vi "valve_shaking - Copy.vi"(0 "Z":T3={"Z_ASw"=1, "Z_HSetState"=enum."on", "Z_ASetState"=enum."on", "Z_DSetState"=enum."on"}, 5 "Y":T1={"Y_ASw"=1, "Y_HSetState"=enum."auto", "Y_ASetState"=enum."auto", "Y_DSetState"=enum."auto"}, 9 "ALR_DI":T2, 12 "Parameters table":u32[](array[numeric])=[0, 10000, 100, 5000, 100, 5000, 1000, 3000]) -> (4 "Z_out":T4, 6 "YB":bool[](array[boolean]), 10 "ALR_ON":bool[](array[boolean]))   [LabVIEW 2015]
uses:
  Userlib.lvlib
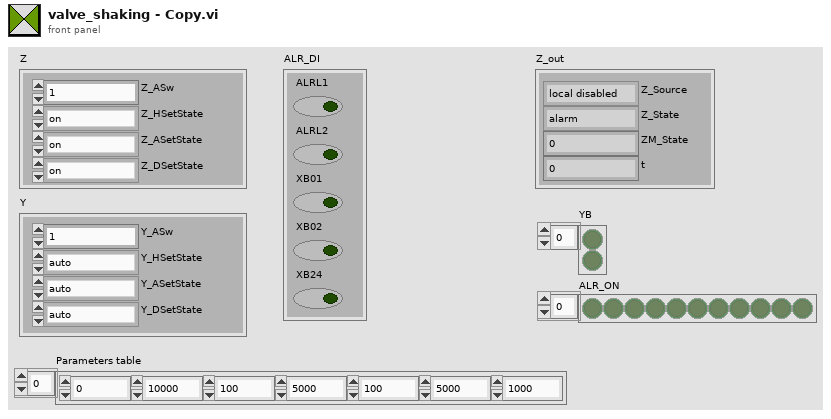
[diagram p1: front panel]
types:
  T1 = cluster{"Y_ASw":u32, "Y_HSetState":enum8{"alarm", "min", "stop", "hand", "auto", "max"}, "Y_ASetState":enum8{"alarm", "min", "stop", "hand", "auto", "max"}, "Y_DSetState":enum8{"alarm", "min", "stop", "hand", "auto", "max"}}
  T2 = cluster{"ALRL1":bool, "ALRL2":bool, "XB01":bool, "XB02":bool, "XB24":bool}
  T3 = cluster{"Z_ASw":u32, "Z_HSetState":enum8{"alarm", "disabled", "not ready", "stop ready", "reserv", "switched off", "switched on", "check", "on min", "decrease speed", "on", "increase speed", "on max"}, "Z_ASetState":enum8{"alarm", "disabled", "not ready", "stop ready", "reserv", "switched off", "switched on", "check", "on min", "decrease speed", "on", "increase speed", "on max"}, "Z_DSetState":enum8{"alarm", "disabled", "not ready", "stop ready", "reserv", "switched off", "switched on", "check", "on min", "decrease speed", "on", "increase speed", "on max"}}
  T4 = cluster{"Z_Source":enum8{"local disabled", "local hand", "hand", "auto", "dist"}, "Z_State":enum8{"alarm", "disabled", "not ready", "stop ready", "reserv", "switched off", "switched on", "check", "on min", "decrease speed", "on", "increase speed", "on max"}, "ZM_State":u8, "t":u32}
  T5 = enum8{"alarm", "disabled", "not ready", "stop ready", "reserv", "switched off", "switched on", "check", "on min", "decrease speed", "on", "increase speed", "on max"}
  T6 = enum8{"local disabled", "local hand", "hand", "auto", "dist"}
  T7 = cluster{"Z_Source_Out":enum8{"local disabled", "local hand", "hand", "auto", "dist"}, "Z_State":enum8{"alarm", "disabled", "not ready", "stop ready", "reserv", "switched off", "switched on", "check", "on min", "decrease speed", "on", "increase speed", "on max"}, "ZM_State":u32, "t":u32}
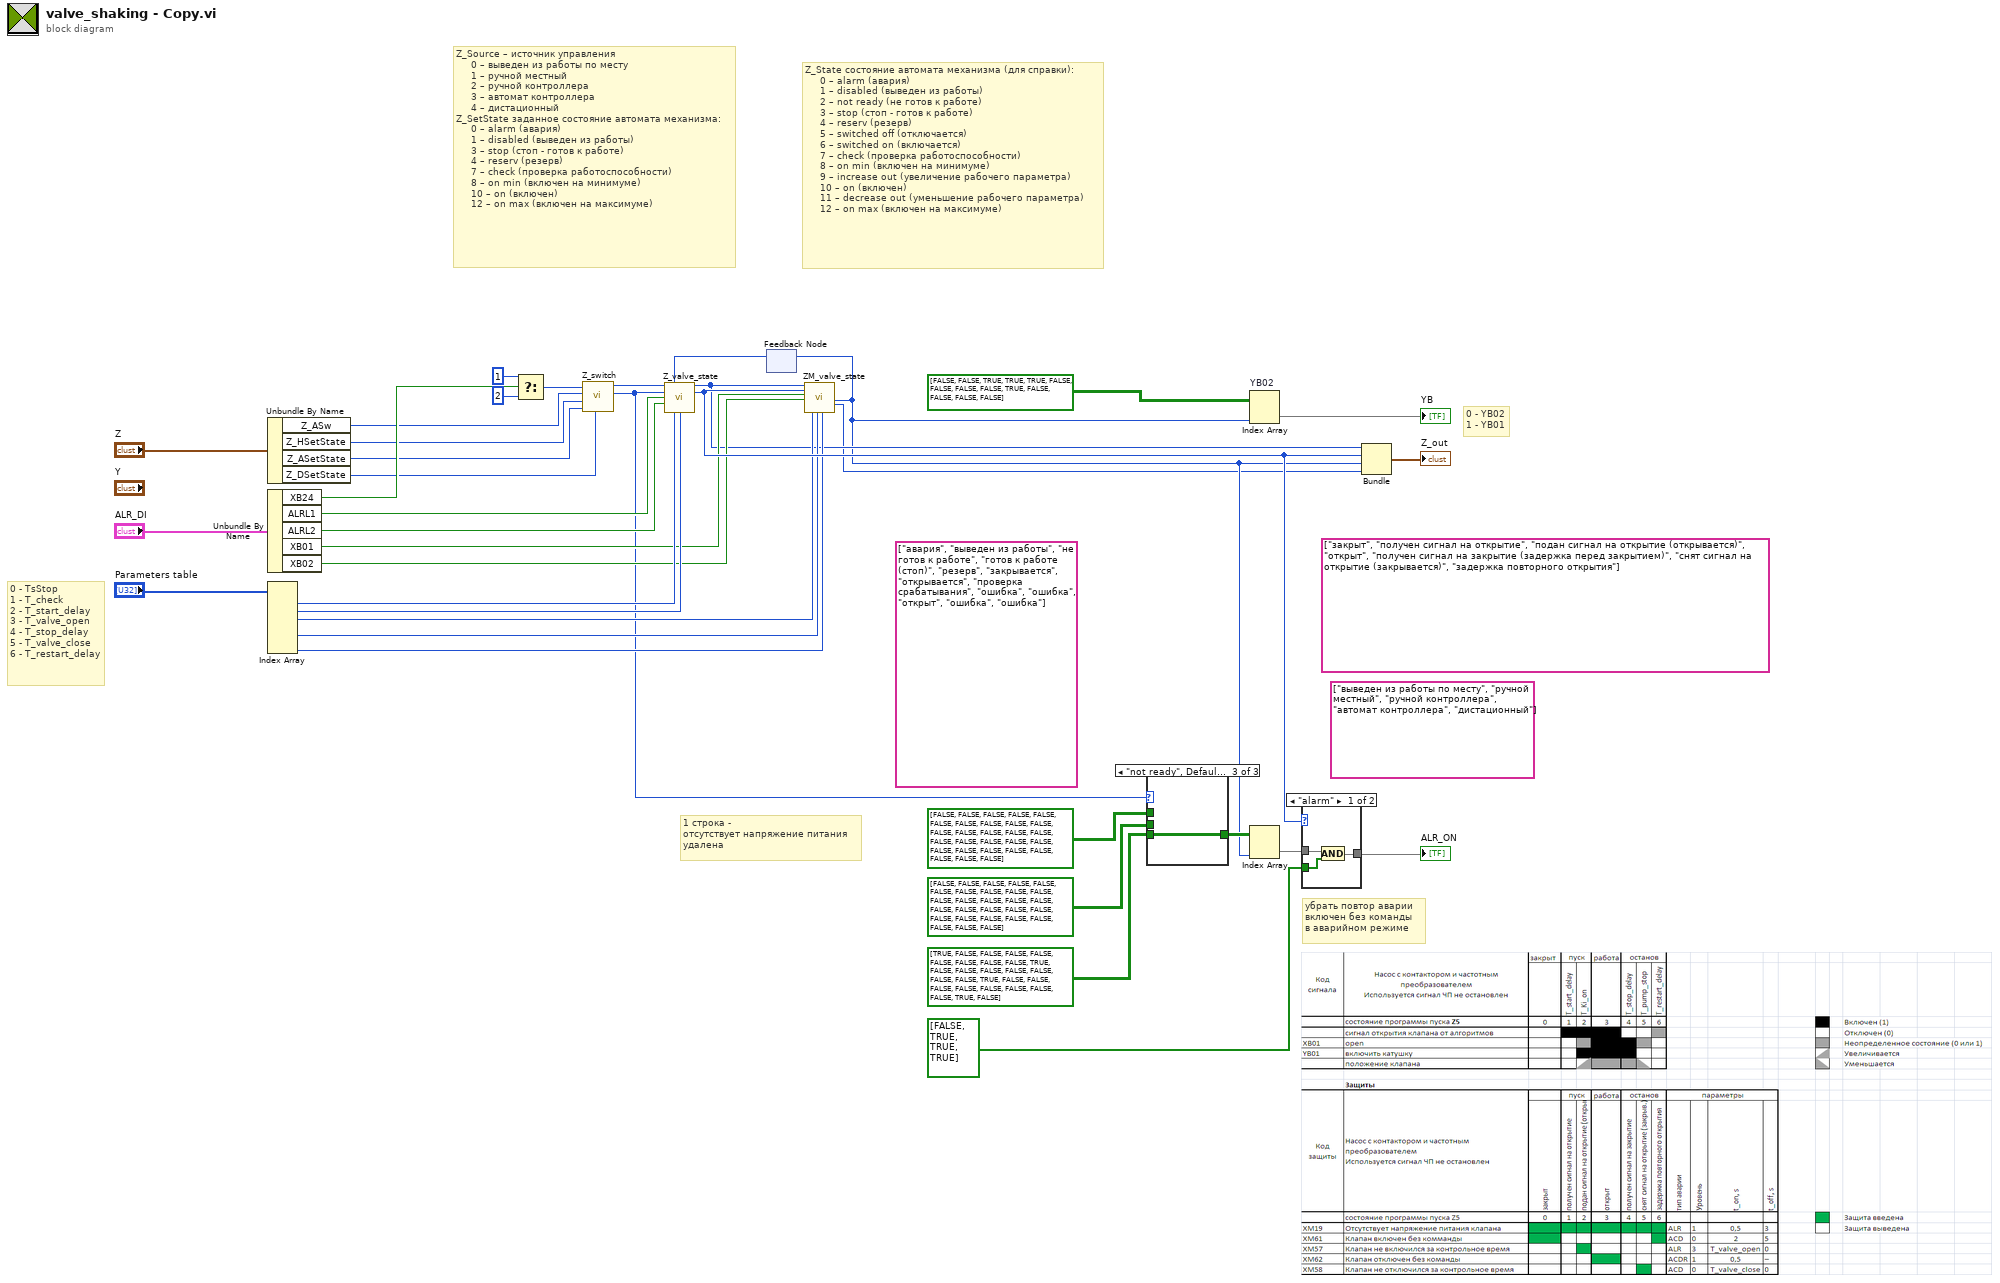
[diagram p0: block diagram]
diagram:
  (unwired) string[] ["закрыт", "получен сигнал на открытие", "подан сигнал на открытие (открывается)", "открыт", "получен сигнал на закрытие (задержка перед закрытием)", "снят сигнал на открытие (закрывается)", "задержка повторного открытия"]
  (unwired) string[] ["выведен из работы по месту", "ручной местный", "ручной контроллера", "автомат контроллера", "дистационный"]
  (unwired) string[] ["авария", "выведен из работы", "не готов к работе", "готов к работе (стоп)", "резерв", "закрывается", "открывается", "проверка срабатывания", "ошибка", "ошибка", "открыт", "ошибка", "ошибка"]
  # "0 - YB02\n1 - YB01"
  # "1 строка - \nотсутствует напряжение питания\nудалена"
  # "убрать повтор аварии\nвключен без команды\nв аварийном режиме"
  # "0 - TsStop\n1 - T_check\n2 - T_start_delay\n3 - T_valve_open\n4 - T_stop_delay\n5 - T_valve_close\n6 - T_restart_delay"
  # "Z_Source – источник управления\n     0 – выведен из работы по месту\n     1 – ручной местный\n     2 – ручной контроллера\n     3 – автомат контроллера\n     4 – дистационный\nZ_SetState заданное состояние автомата механизма:\n     0 – alarm (авария)\n     1 – disabled (выведен из работы)\n     3 – stop (стоп - готов к работе)\n     4 – reserv (резерв)\n     7 – check (проверка работоспособности)\n     8 – on min (включен на минимуме)\n     10 – on (включен)\n     12 – on max (включен на максимуме)"
  # "Z_State состояние автомата механизма (для справки):\n     0 – alarm (авария)\n     1 – disabled (выведен из работы)\n     2 – not ready (не готов к работе)\n     3 – stop (стоп - готов к работе)\n     4 – reserv (резерв)\n     5 – switched off (отключается)\n     6 – switched on (включается)\n     7 – check (проверка работоспособности)\n     8 – on min (включен на минимуме)\n     9 – increase out (увеличение рабочего параметра)\n     10 – on (включен)\n     11 – decrease out (уменьшение рабочего параметра)\n     12 – on max (включен на максимуме)"
  n1 = Unbundle By Name("Z") -> ("Z_ASw"=w11:u32, "Z_HSetState"=w8:T5, "Z_ASetState"=w7:T5, "Z_DSetState"=w6:T5)
  n2 = Unbundle By Name("ALR_DI") -> ("XB24"=w12:bool, "ALRL1"=w16:bool, "ALRL2"=w15:bool, "XB01"=w14:bool, "XB02"=w13:bool)
  n3 = Index Array(array="Parameters table") -> (element #1=w32:u32, element #2=w24:u32, element #3=w19:u32, element #5=w18:u32, element #7=w17:u32)  [unwired: 7 in, 2 out]
  n4 = Select(t=u32 1, s=w12, f=u32 2) -> (s? t:f=w33:u32)
  n5 = call "Z_switch.vi"("Z_DSetState"=w6, "Z_ASetState"=w7, "Z_HSetState"=w8, "Z_ASw"=w11, "Z_HSw"=w33) -> ("Z_SetState"=w9:T5, "Z_Source"=w10:T6)  [unwired: 5 in]
  n6 = feedback #1() -> (w34:u32)  [unwired: 1 in]
  n7 = call "Z_valve_state.vi"("Z_Source"=w10, "ZM_State"=w34, "Z_SetState"=w9, "Alarm_L1"=w16, "Alarm_L2"=w15, "TsStop"=w32, "t_check"=w24) -> ("Z_Source_Out"=w5:T6, "Z_State"=w23:T5)  [unwired: 6 in, 1 out]
  n8 = call "ZM_valve_state.vi"("Z_Source"=w5, "Z_State"=w23, "open"=w14, "close"=w13, "T_start_delay"=w19, "T_stop_delay"=w18, "T_restart_delay"=w17) -> ("ZM_State"=w4:u32, "t"=w2:u32)  [unwired: 8 in, 3 out]
  n9 = feedback-in #1(w4) -> ()
  n10 = case shown="\"not ready\", Default" w9 {
    tunnel: bool[][] [[FALSE, FALSE, FALSE, FALSE, FALSE, FALSE, FALSE], [FALSE, FALSE, FALSE, FALSE, FALSE, FALSE, FALSE], [FALSE, FALSE, FALSE, FALSE, FALSE, FALSE, FALSE], [FALSE, FALSE, FALSE, FALSE, FALSE, FALSE, FALSE]] ("Array") -> [w38 _ _]
    tunnel: bool[][] [[FALSE, FALSE, FALSE, FALSE, FALSE, FALSE, FALSE], [FALSE, FALSE, FALSE, FALSE, FALSE, FALSE, FALSE], [FALSE, FALSE, FALSE, FALSE, FALSE, FALSE, FALSE], [FALSE, FALSE, FALSE, FALSE, FALSE, FALSE, FALSE]] ("Array 2") -> [_ w39 _]
    tunnel: bool[][] [[TRUE, FALSE, FALSE, FALSE, FALSE, FALSE, FALSE], [FALSE, FALSE, TRUE, FALSE, FALSE, FALSE, FALSE], [FALSE, FALSE, FALSE, TRUE, FALSE, FALSE, FALSE], [FALSE, FALSE, FALSE, FALSE, FALSE, TRUE, FALSE]] ("Array 3") -> [_ _ w40]
    tunnel: [w38 w39 w40] -> w28
    frame "alarm" {
    }
    frame "disabled" {
    }
    frame "not ready", Default {
    }
  }
  n11 = Index Array "YB02"(array=bool[][] [[FALSE, FALSE, TRUE, TRUE, TRUE, FALSE, FALSE], [FALSE, FALSE, TRUE, FALSE, FALSE, FALSE, FALSE]] ("Array 5"), index (col)=w4) -> (element=→"YB":bool[])  [unwired: 1 in]
  n12 = Index Array(array=w28, index (col)=w4) -> (element=w26:bool[])  [unwired: 1 in]
  n13 = case shown="\"alarm\"" w23 {
    tunnel: bool[] [FALSE, TRUE, TRUE, TRUE] ("Array 4") -> [w42 _]
    tunnel: w26 -> [w43 w44]
    tunnel: [w41 w44] -> w25
    frame "alarm" {
      n14 = And(x=w43, y=w42) -> (x .and. y?=w41:bool[])
    }
    frame "disabled", Default {
    }
  }
  "ALR_ON" <- w25
  n15 = Bundle("Z_Source_Out"=w5, "Z_State"=w23, "ZM_State"=w4, "t"=w2) -> (→"Z_out":T7)  [unwired: 1 in]
